vi "Write Standard Config.vi"(8 "error in (no error)":errorcluster, 11 "CCDCamera in":refnum<class "CCDCamera.lvclass">) -> (0 "error out":errorcluster, 3 "CCDCamera out":refnum<class "CCDCamera.lvclass">)   [LabVIEW 2018, in "CCDCamera.lvclass"]
doc: "This VI writes a standar configuration to the class."
uses:
  CCDCamera.lvclass
  CCDCamera.lvclass/CCDCamera.ctl
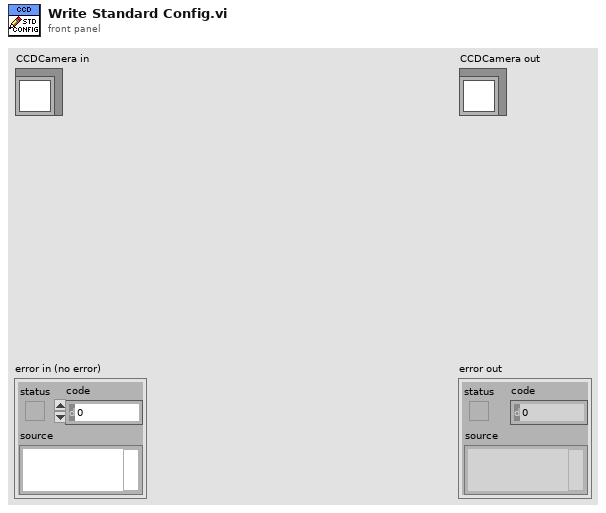
[diagram p1: front panel]
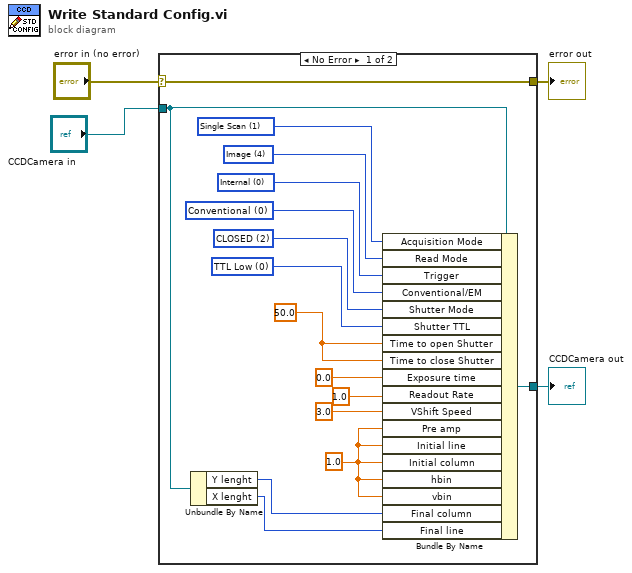
[diagram p0: block diagram]
diagram:
  n1 = case shown="No Error" "error in (no error)" {
    selector: "error in (no error)" -> [w20 w22]
    tunnel: [w20 w22] -> w3
    tunnel: [w19 w21] -> w1
    tunnel: "CCDCamera in" -> [w10 w21]
    frame No Error {
      w7 = 1.0 ("hbin")
      w9 = 50.0 ("Time to close Shutter")
      w18 = u16 0 items=["TTL Low", "TTL High"] ("Shutter TTL")
      w16 = u16 2 items=["Fully Auto", "OPEN", "CLOSED"] ("Shutter Mode")
      w15 = u16 0 items=["Conventional", "EM Gain"] ("Conventional/EM")
      w14 = u16 0 items=["Internal", "External", "N/A", "N/A", "N/A", "N/A", "External Start", "External Exposure (bulb)", "N/A", "External FVB EM", "Software", "N/A", "External Charge Shifting"] ("Trigger")
      w13 = u16 4 items=["Full Vertical Binning", "Multi-Track", "Random-Track", "Single-Track", "Image"] ("Read Mode")
      w12 = u16 1 items=["RESERVED", "Single Scan", "Accumulate", "Kinetics", "Fast Kinetics", "Run Til Abort", "RESERVED", "RESERVED", "RESERVED", "RESERVED", "Time Delayed Integration"] ("Acquisition Mode")
      n2 = Unbundle By Name(w10) -> ("Y lenght"=w5:u16, "X lenght"=w6:u16)
      n3 = Bundle By Name(cluster=w10, "Acquisition Mode"=w12, "Read Mode"=w13, "Trigger"=w14, "Conventional/EM"=w15, "Shutter Mode"=w16, "Shutter TTL"=w18, "Time to open Shutter"=w9, "Time to close Shutter"=w9, "Exposure time"=0.0 ("Y lenght"), "Readout Rate"=1.0 ("hbin"), "VShift Speed"=3.0, "Pre amp"=w7, "Initial line"=w7, "Initial column"=w7, "hbin"=w7, "vbin"=w7, "Final column"=w5, "Final line"=w6) -> (w19:refnum<class "CCDCamera.lvclass">)
    }
    frame Error {
    }
  }
  "error out" <- w3
  "CCDCamera out" <- w1
